vi "Get max deflection and Zpos index value.vi"(0 "reference in":refnum<class "Fcurve.lvclass">, 1 ">Zpos (V): Sensor IN>":dbl[](array[numeric]), 2 ">Deflection (V)>":dbl[](array[numeric]), 5 "error in (no error)":errorcluster) -> (14 "reference out":refnum<class "Fcurve.lvclass">, 19 "error out":errorcluster)   [LabVIEW 2019]
doc: "Gets the deflection (V) array, searches for the (Max value) index and corresponding values"
uses:
  Fcurve.lvclass
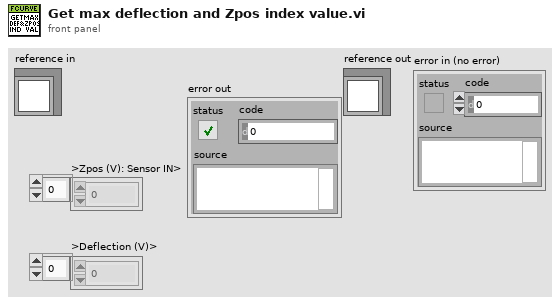
[diagram p1: front panel]
types:
  T1 = typedef "Fcurve.lvclass/ObjectAttributesRef.ctl" = refnum<data-value>
  T2 = typedef "Fcurve.lvclass/ObjectAttributes.ctl" = cluster{"MyAttribute":dbl, "Fcurve Metadata":T3, "Contact Spread of dev":dbl, "Tau Delay (ms)":dbl, "Points of contact":dbl, "Def_wfm":cluster{"Max":dbl, "Min":dbl}, "Zpos_wfm":cluster{"Max":dbl, "Min":dbl}, "Contact stat?":bool, "Real AI dt (s)":dbl, "Decimation":cluster{"App":cluster{"Dec":i32, "apply":bool}, "Con":cluster{"Dec":i32, "apply":bool}, "Ret":cluster{"Dec":i32, "apply":bool}}, "Segment def[0]":dbl, "Segment Zpos[0]":dbl, "Raw Datum":waveform(dbl)[], "Group metadata":T4, "M_data obj":refnum<class "metadata.lvclass">, "Channel name(s)":string[], "Segment fcurve data":cluster{"X":dbl[], "Y":dbl[]}[], "Segment duration":cluster{"Start":i32, "Duration":i32}[], "Segment info":T5[], "Segment durations (S)":dbl[], "Segments Maxmin":T7[]}
  T3 = typedef "Fcurve.lvclass/Metadata.ctl" = cluster{"dt (us)":dbl, "Dec Factor":dbl, "Z piezo Sensitivity (nm/V)":dbl, "K (N/m)":dbl, "Sp (V)":dbl, "Contact (ms)":dbl, "Zpos contact":dbl, "Vel_app (nm/s)":dbl, "Vel_ret (nm/s)":dbl, "deltaV (nm)":dbl, "Def_V0 (v)":dbl, "Piezo gain":dbl, "invOLS (nm/V)":dbl}
  T4 = typedef "TDMS_DataHandler.lvclass/Fcurve Meta data.ctl" = cluster{"property names":string[], "property values":variant[]}
  T5 = typedef "Fcurve.lvclass/Fcurve segments --cluster.ctl" = cluster{"type":T6, "nb points":i32, "dec factor":u32, "sampling rate (S/s)":u32}
  T6 = typedef "metadata.lvclass/Segment type--combobox.ctl" = string
  T7 = typedef "Fcurve.lvclass/Segment MaxMin --cluster.ctl" = cluster{"Def":cluster{"max value":dbl, "min value":dbl}, "Zpos":cluster{"max value":dbl, "min value":dbl}}
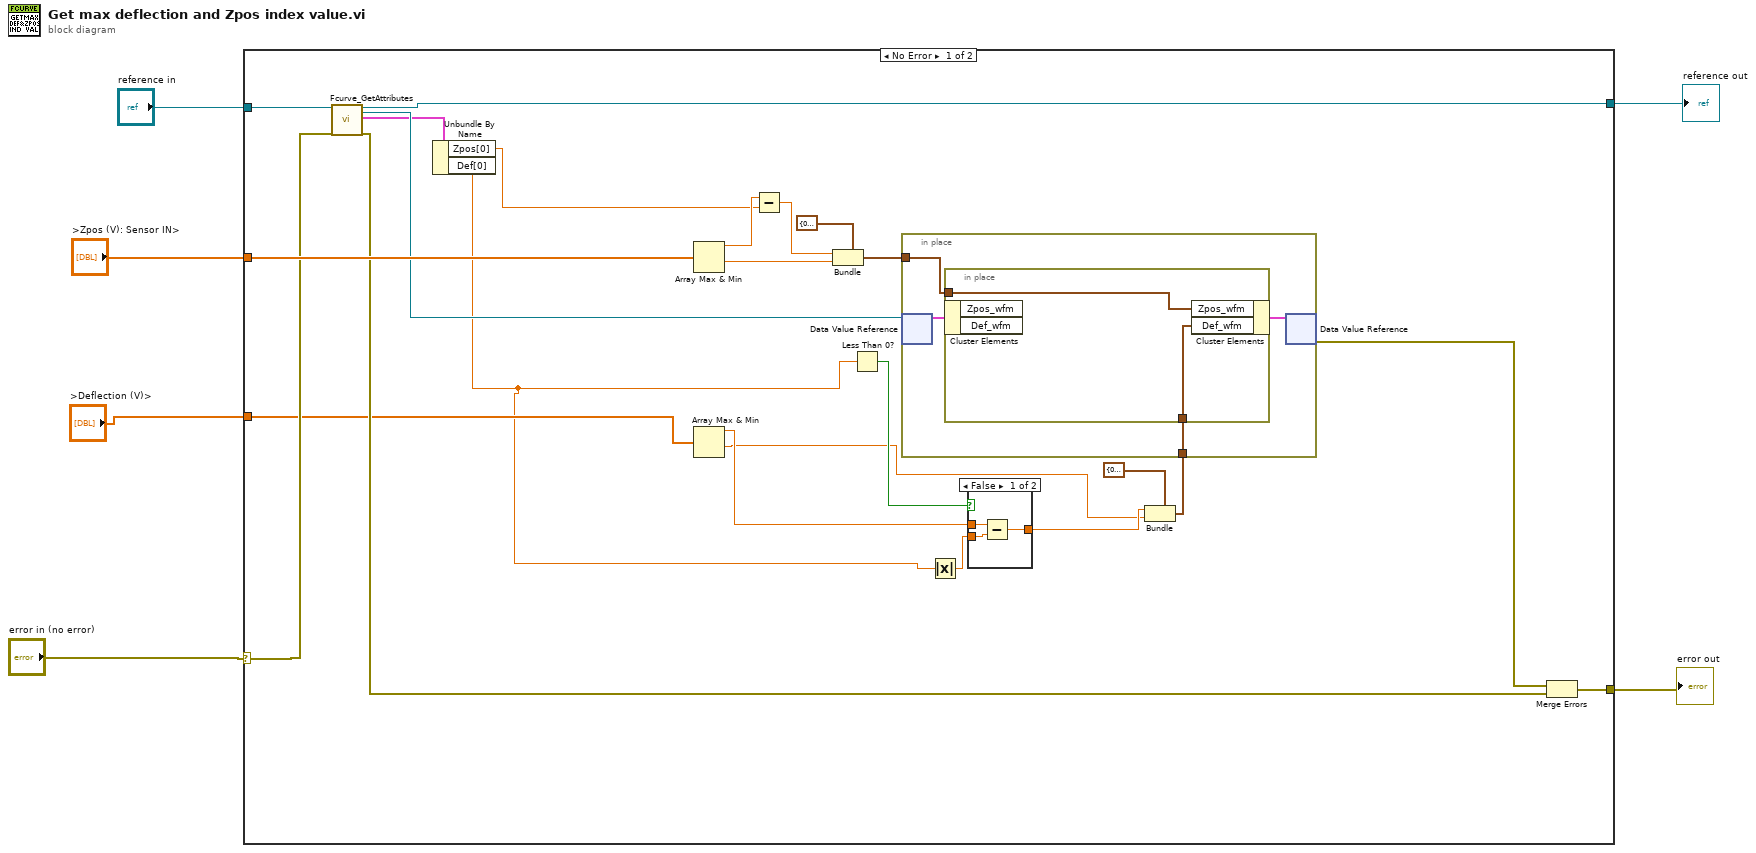
[diagram p0: block diagram]
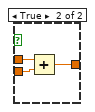
[diagram p2: hidden frame]
diagram:
  n1 = case shown="No Error" "error in (no error)" {
    selector: "error in (no error)" -> [w18 w43]
    tunnel: ">Zpos (V): Sensor IN>" -> [w25 _]
    tunnel: "reference in" -> [w23 w44]
    tunnel: [w21 w43] -> w4
    tunnel: [w20 w44] -> w3
    tunnel: ">Deflection (V)>" -> [w15 _]
    frame No Error {
      n2 = call "Fcurve_GetAttributes.vi"("reference in"=w23, "error in (no error)"=w18) -> ("reference out"=w20:refnum<class "Fcurve.lvclass">, "attributes ref"=w24:T1, "attributes"=w17:T2, "error out"=w19:errorcluster)  [unwired: 14 in]
      n3 = Unbundle By Name(w17) -> ("Zpos[0]"=w16:dbl, "Def[0]"=w12:dbl)
      n4 = Array Max & Min(array=w25) -> (max value=w28:dbl, min value=w27:dbl)  [unwired: 2 out]
      n5 = Array Max & Min(array=w15) -> (max value=w13:dbl, min value=w8:dbl)  [unwired: 2 out]
      n6 = Subtract(x=w28, y=w16) -> (x-y=w29:dbl)
      n7 = Bundle(cluster=cluster{"Max":dbl, "Min":dbl} {"Max"=0.0, "Min"=0.0} ("Zpos"), "Max"=w29, "Min"=w27) -> (w30:cluster{"Max":dbl, "Min":dbl})
      n8 = Less Than 0?(x=w12) -> (x < 0?=w11:bool)
      n9 = Absolute Value(x=w12) -> (abs(x)=w14:dbl)
      n10 = case shown="False" w11 {
        tunnel: w13 -> [w33 w36]
        tunnel: w14 -> [w32 w35]
        tunnel: [w31 w34] -> w9
        frame False {
          n11 = Subtract(x=w33, y=w32) -> (x-y=w31:dbl)
        }
        frame True {
          n12 = Add(x=w36, y=w35) -> (x+y=w34:dbl)
        }
      }
      n13 = Bundle(cluster=cluster{"Max":dbl, "Min":dbl} {"Max"=0.0, "Min"=0.0} ("Def_wfm"), "Max"=w9, "Min"=w8) -> (w7:cluster{"Max":dbl, "Min":dbl})
      n14 = in-place {
        in-place-border: w30 -> [w38]
        in-place-border: w7 -> [w37]
        n15 = in-place-dvr #1(w24) -> (w39:T2)  [unwired: 1 out]
        n16 = in-place {
          in-place-border: w38 -> [w42]
          in-place-border: w37 -> [w41]
          n17 = in-place-cluster #2(w39) -> ()  [unwired: 2 out]
          n18 = in-place-cluster #2("Zpos_wfm"=w42, "Def_wfm"=w41) -> (w40:T2)
        }
        n19 = in-place-dvr #1(w40) -> (w22:errorcluster)  [unwired: 1 out]
      }
      n20 = Merge Errors(w22, w19) -> (w21:errorcluster)
    }
    frame Error {
    }
  }
  "error out" <- w4
  "reference out" <- w3
